vi "DecodePulse.vi"(10 "ValidInput":bool, 11 "OnTime":u32) -> (2 "OutputValid":bool, 3 "s? t:f":T1=enum."Marker")   [LabVIEW 2019]
uses:
  TypeDefs/TimeSymbol.ctl
panel:
  in  "OffTime":u32
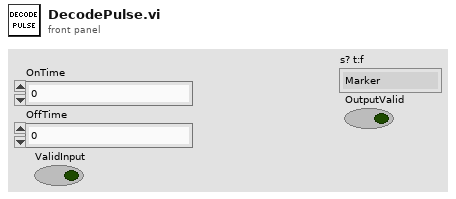
[diagram p1: front panel]
types:
  T1 = typedef "TimeSymbol.ctl" = enum16{"0", "1", "Marker", "Invalid"}
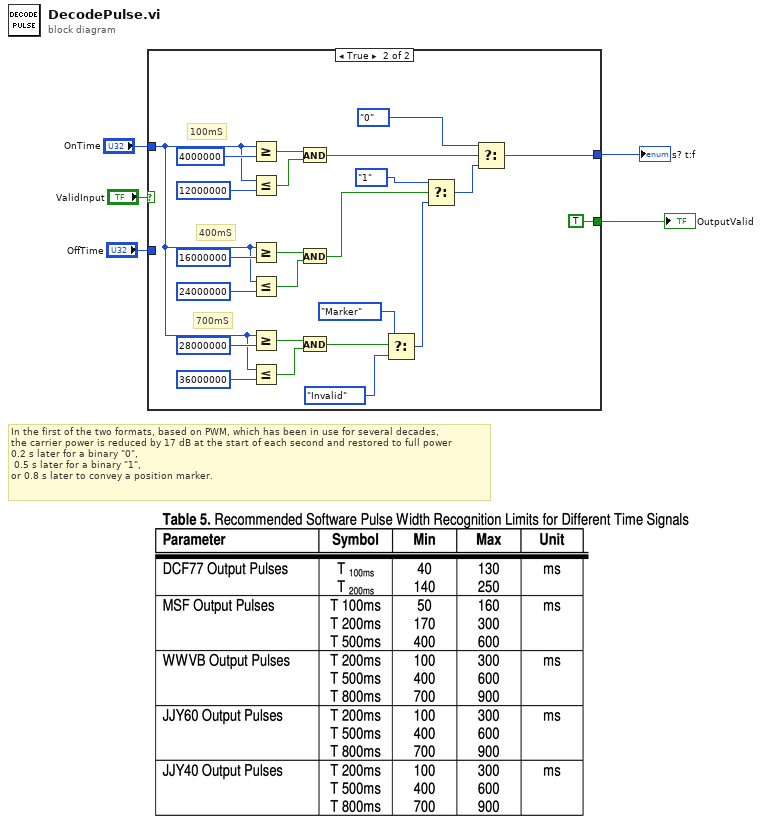
[diagram p0: block diagram]
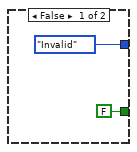
[diagram p2: hidden frame]
diagram:
  # "In the first of the two formats, based on PWM, which has been in use for several decades, \nthe carrier power is reduced by 17 dB at the start of each second and restored to full power \n0.2 s later for a binary \"0\",\n 0.5 s later for a binary \"1\", \nor 0.8 s later to convey a position marker."
  n1 = case shown="True" "ValidInput" {
    tunnel: "OnTime" -> [_ w19]
    tunnel: "OffTime" -> [_ _]
    tunnel: [TimeSymbol."Invalid" w9] -> w2
    tunnel: [FALSE ("OutputValid") TRUE ("OutputValid")] -> w1
    frame False {
    }
    frame True {
      # "700mS"
      # "400mS"
      # "100mS"
      n2 = Greater Or Equal?(x=w19, y=u32 4000000) -> (x >= y?=w30:bool)
      n3 = Less Or Equal?(x=w19, y=u32 12000000) -> (x <= y?=w28:bool)
      n4 = Greater Or Equal?(x=w19, y=u32 16000000) -> (x >= y?=w26:bool)
      n5 = Less Or Equal?(x=w19, y=u32 24000000) -> (x <= y?=w24:bool)
      n6 = Greater Or Equal?(x=w19, y=u32 28000000) -> (x >= y?=w22:bool)
      n7 = Less Or Equal?(x=w19, y=u32 36000000) -> (x <= y?=w20:bool)
      n8 = And(x=w30, y=w28) -> (x .and. y?=w18:bool)
      n9 = And(x=w26, y=w24) -> (x .and. y?=w15:bool)
      n10 = And(x=w22, y=w20) -> (x .and. y?=w11:bool)
      n11 = Select(t=TimeSymbol."Marker", s=w11, f=TimeSymbol."Invalid") -> (s? t:f=w13:T1)
      n12 = Select(t=TimeSymbol."1", s=w15, f=w13) -> (s? t:f=w16:T1)
      n13 = Select(t=TimeSymbol."0", s=w18, f=w16) -> (s? t:f=w9:T1)
    }
  }
  "s? t:f" <- w2
  "OutputValid" <- w1
